vi "bold_text_lines.vi"(8 "error in (no error)":errorcluster, 10 "Lines to bold":i32[](array[numeric]), 11 "String to bold reference":refnum<vi>) -> (0 "error out":errorcluster)   [LabVIEW 2020]
panel:
  # "Inputs"
  # "Outputs"
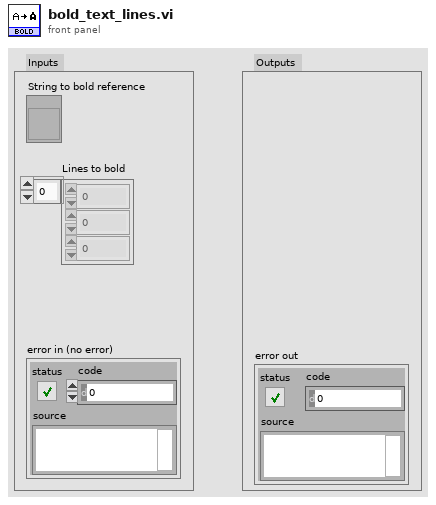
[diagram p1: front panel]
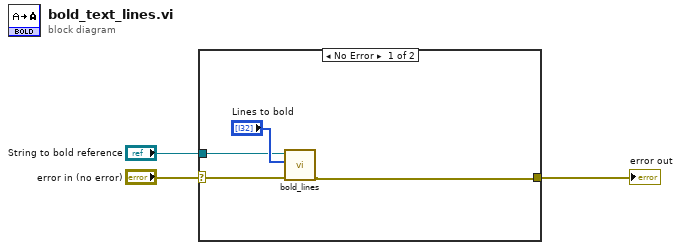
[diagram p0: block diagram]
diagram:
  n1 = case shown="No Error" "error in (no error)" {
    selector: "error in (no error)" -> [w5 w8]
    tunnel: "String to bold reference" -> [w6 _]
    tunnel: [w4 w8] -> w1
    frame No Error {
      n2 = call "bold_lines.vi"("error in (no error)"=w5, "Lines to bold"="Lines to bold", "String reference in"=w6) -> ("error out"=w4:errorcluster)  [unwired: 7 in, 1 out]
    }
    frame Error {
    }
  }
  "error out" <- w1
